vi "Test_String_Publish_Observe_ValueOK.vi"(8 "error in (no error)":errorcluster, 11 "TestCase in":refnum<class "TestObservableDataTypes.lvclass">) -> (0 "error out":errorcluster, 3 "TestCase out":refnum<class "TestObservableDataTypes.lvclass">)   [LabVIEW 2017, in "TestObservableDataTypes.lvclass"]
uses:
  TestObservableDataTypes.lvclass
  Source/Framework/Mediator/Mediator/Mediator.lvclass
  C:/Program Files (x86)/National Instruments/LabVIEW 2017/vi.lib/ActorFramework/Actor/Actor.lvclass
  Source/Framework/IMediator/PublishRequest/PublishRequest.lvclass/PublishRequest.ctl
  Source/Framework/SubscriptionPolicy/BasicSubscription/BasicSubscription.lvclass/BasicSubscription.ctl
  gpm_packages/@cs/transport/Source/Concrete/NotifierTransport/NotifierTransport.lvclass/NotifierTransport.ctl
  Source/Framework/IMediator/SubscriptionRequest/SubscriptionRequest.lvclass/SubscriptionRequest.ctl
  Source/Framework/IMediator/IMediator Messages/Subscribe Msg/Subscribe Msg.lvclass/Subscribe Msg.ctl
  <vilib>/ActorFramework/Message Enqueuer/Message Enqueuer.lvclass/Message Enqueuer.ctl
  Source/Framework/IMediator/IMediator Messages/Publish Msg/Publish Msg.lvclass/Publish Msg.ctl
  <vilib>/ActorFramework/Message Enqueuer/Enqueue.vi
  Source/Framework/SubscriptionPolicy/BasicSubscription/BasicSubscription.lvclass
  C:/Git/mva-framework/Source/Framework/IMediator/ISubscriptionPolicy/ISubscriptionPolicy.lvclass
  gpm_packages/@cs/transport/Source/Concrete/NotifierTransport/NotifierTransport.lvclass
  C:/Git/mva-framework/gpm_packages/@cs/transport/Source/ITransport/ITransport.lvclass
  Source/Framework/IMediator/IMediator Messages/Subscribe Msg/Subscribe Msg.lvclass
  C:/Program Files (x86)/National Instruments/LabVIEW 2017/vi.lib/ActorFramework/Message/Message.lvclass
  Source/Framework/IMediator/IMediator Messages/Publish Msg/Publish Msg.lvclass
  <vilib>/ActorFramework/Stop Msg/Stop Msg.lvclass
  <vilib>/ActorFramework/Message Priority Queue/Priority Enqueue.vi
  <vilib>/Utility/error.llb/Error Cluster From Error Code.vi
  Source/Framework/IMediator/SubscriptionRequest/SubscriptionRequest.lvclass
  Source/Framework/IMediator/PublishRequest/PublishRequest.lvclass
  Source/Framework/IMediator/ISubscriptionPolicy/ISubscriptionPolicy.lvclass
  <vilib>/ActorFramework/Actor/Actor.lvclass
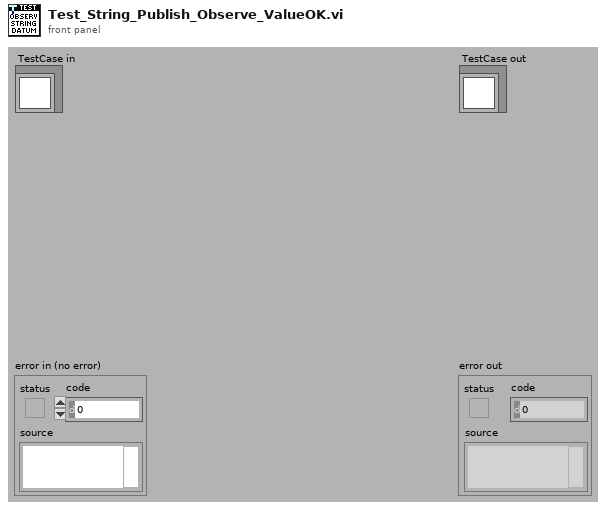
[diagram p1: front panel]
types:
  T1 = typedef "IMediator.lvlib/ISubscriptionPolicy.lvclass/ISubscriptionPolicy Reference.ctl" = refnum<data-value>
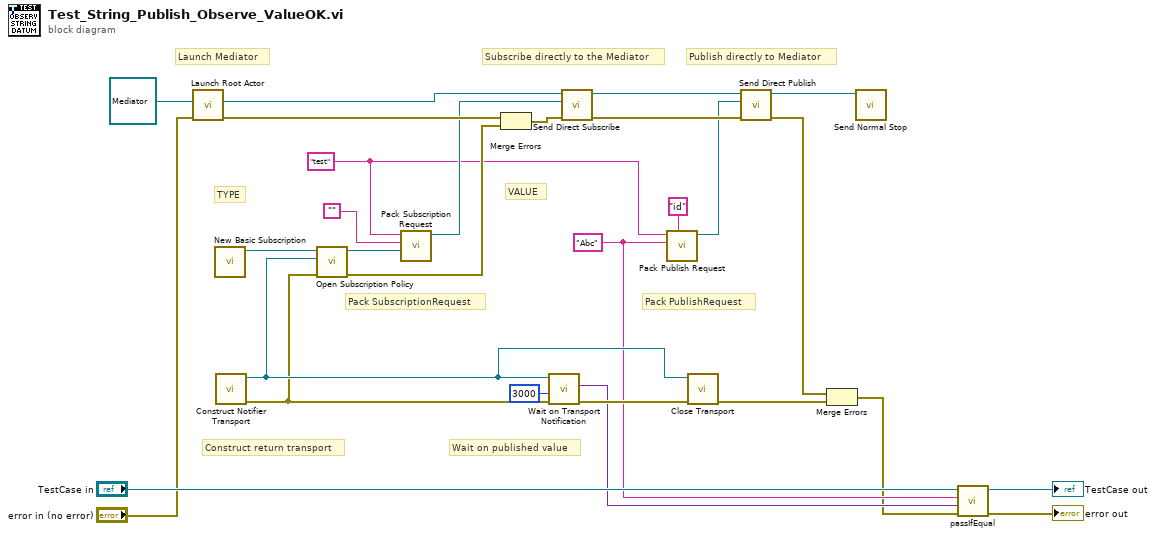
[diagram p0: block diagram]
diagram:
  w5 = "Abc"
  w11 = "test" ("Topic Name")
  # "VALUE"
  # "TYPE"
  # "Construct return transport"
  # "Wait on published value"
  # "Publish directly to Mediator"
  # "Pack PublishRequest"
  # "Launch Mediator"
  # "Pack SubscriptionRequest"
  # "Subscribe directly to the Mediator"
  n1 = call <vilib>:"Launch Root Actor.vi"("error in (no error)"="error in (no error)", "Actor"=refnum<class "Mediator.lvclass"> refnum ("Mediator.lvlib:Mediator.lvclass")) -> ("error out"=w17:errorcluster, "Actor's Enqueuer"=w20:refnum<class "Message Enqueuer.lvclass">)  [unwired: 8 in]
  n2 = call "New Basic Subscription.vi"() -> ("BasicSubscription Out"=w24:refnum<class "BasicSubscription.lvclass">)  [unwired: 11 in]
  n3 = call "Construct Notifier Transport.vi"() -> ("error out"=w3:errorcluster, "NotifierTransport"=w10:refnum<class "NotifierTransport.lvclass">)  [unwired: 10 in]
  n4 = call "Open Subscription Policy.vi"("error in (no error)"=w3, "Transport"=w10, "SubscriptionPolicy"=w24) -> ("error out"=w14:errorcluster, "Subscription Policy"=w23:T1)  [unwired: 7 in]
  n5 = call "Pack Subscription Request.vi"("Subscription Policy"=w23, "Type"="", "Datum Name"=w11) -> ("SubscriptionRequest"=w16:refnum<class "SubscriptionRequest.lvclass">)  [unwired: 8 in]
  n6 = Merge Errors(w17, w14) -> (w15:errorcluster)
  n7 = call "Wait on Transport Notification.vi"("error in (no error)"=w3, "Timeout In ms (-1)"=3000, "NotifierTransport"=w10) -> ("error out"=w7:errorcluster, "Data"=w6:variant)  [unwired: 6 in, 1 out]
  n8 = call "Send Direct Subscribe.vi"("error in (no error)"=w15, "Subscription Request"=w16, "Message Enqueuer"=w20) -> ("error out"=w9:errorcluster, "Message Enqueuer out"=w19:refnum<class "Message Enqueuer.lvclass">)  [unwired: 7 in]
  n9 = call "Pack Publish Request.vi"("Publisher ID"="id", "Data to Publish"=w5, "Datum Name"=w11) -> ("PublishRequest"=w8:refnum<class "PublishRequest.lvclass">)  [unwired: 8 in]
  n10 = call-dynamic "Close Transport.vi"("error in (no error)"=w7, "NotifierTransport"=w10) -> ("error out"=w1:errorcluster)  [unwired: 9 in]
  n11 = call "Send Direct Publish.vi"("error in (no error)"=w9, "PublishRequest"=w8, "Mediator Enqeuer"=w19) -> ("error out"=w4:errorcluster, "Mediator Enqueuer out"=w13:refnum<class "Message Enqueuer.lvclass">)  [unwired: 7 in]
  n12 = Merge Errors(w4, w1) -> (w2:errorcluster)
  n13 = call <vilib>:"Send Normal Stop.vi"("Message Enqueuer"=w13) -> ()  [unwired: 10 in, 1 out]
  n14 = call-dynamic "passIfEqual.vi"("error in (no error)"=w2, "y"=w6, "x"=w5, "TestCase in"="TestCase in") -> ("error out"=→"error out":errorcluster, "TestCase out"=→"TestCase out":refnum<class "TestObservableDataTypes.lvclass">)  [unwired: 6 in]
